vi "Topo & GridSpectr_DriftCorrection_v6.vi"(6 "Internal use":string, 7 "Grid param":T2 {"height (m)" format="%#_6p"; "width (m)" format="%#_6p"; "center Y (m)" format="%#_6p"; "center X (m)" format="%#_6p"}, 8 "Error in (no error)":errorcluster, 9 "Points Y/Index Y":i32, 10 "Points X/Index X":i32, 11 "Method":enum16{"init", "run", "end"}(ring)=enum."end") -> (0 "Error out":errorcluster)   [LabVIEW 2014]
doc: "Example of a measurement VI to be used in the \"Experiments on a Grid\" tool as external VI.\n\nThis example measure the topography and spectroscopy data. The spectroscopy measurements are taken on a subgrid. The data are saved to a sxm and a binary file.\n\n- Nanonis Programming Interface -"
uses:
  <userlib>/Nanonis Prog Interface V5/Nanonis Prog Interface.lvlib
panel:
  out "Images taken":i32=14
  in  "increment":i32=16
  in  "trigger":i32=3 min=1 step=1
  in  "tip Speed (m/s)":sgl=1e-08 format="%.2p"
  in  "Drift Correction 2":T1
  out "X drift":i32
  out "Y drift":i32
  out "Queue Steps":i32=40
  in  "StepsBack":i32=40
  in  "Channel index (0-23)":u8=14
  in  "File name":string="single_mol_shortSTS"
  in  "STS Current":dbl=9.999999717180685e-10 format="%#_6p"
  in  "Imaging Current":dbl=5.00000006675716e-11 format="%#_6p"
  in  "zdrift \nDuration (s)":dbl
  in  "Correct z drift":bool
  out "Status":string="finishing"
  in  "Drift correction Pixels":i32=256 caption="Pixels for drift correction"
  out "Y Offset":dbl
  out "X Offset":dbl
  out "Points taken":dbl=14.0
  in  "Drift Correction every":i32=16
  in  "Y subgrid spacing":u16=1
  in  "X subgrid spacing":u16=1
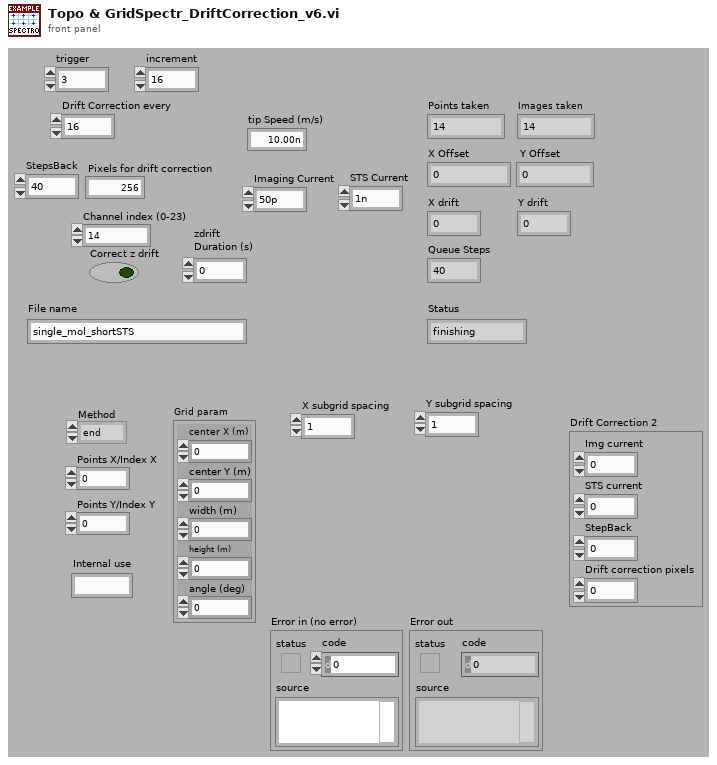
[diagram p1: front panel]
types:
  T1 = cluster{"Img current":dbl, "STS current":dbl, "StepBack":dbl, "Drift correction pixels":dbl}
  T2 = cluster{"center X (m)":sgl, "center Y (m)":sgl, "width (m)":sgl, "height (m)":sgl, "angle (deg)":sgl}
  T3 = cluster{"center X":sgl, "center Y":sgl, "angle":sgl, "width":sgl, "height":sgl, "# pixels":i32, "# lines":i32}
  T4 = cluster{"Name":string, "Calibration":sgl, "Offset":sgl, "Channel index":i32}[]
  T5 = cluster{"up/down":bool, "time/line":sgl, "start time":timestamp, "end time":timestamp}
  T6 = cluster{"Z averaging time (s)":sgl, "Z offset (m)":sgl, "Initial settling time (s)":sgl}
  T7 = cluster{"Max. slew rate (V/s)":sgl, "Settling time (s)":sgl, "Integration time (s)":sgl}
  T8 = cluster{"End settling time (s)":sgl, "Z control time (s)":sgl}
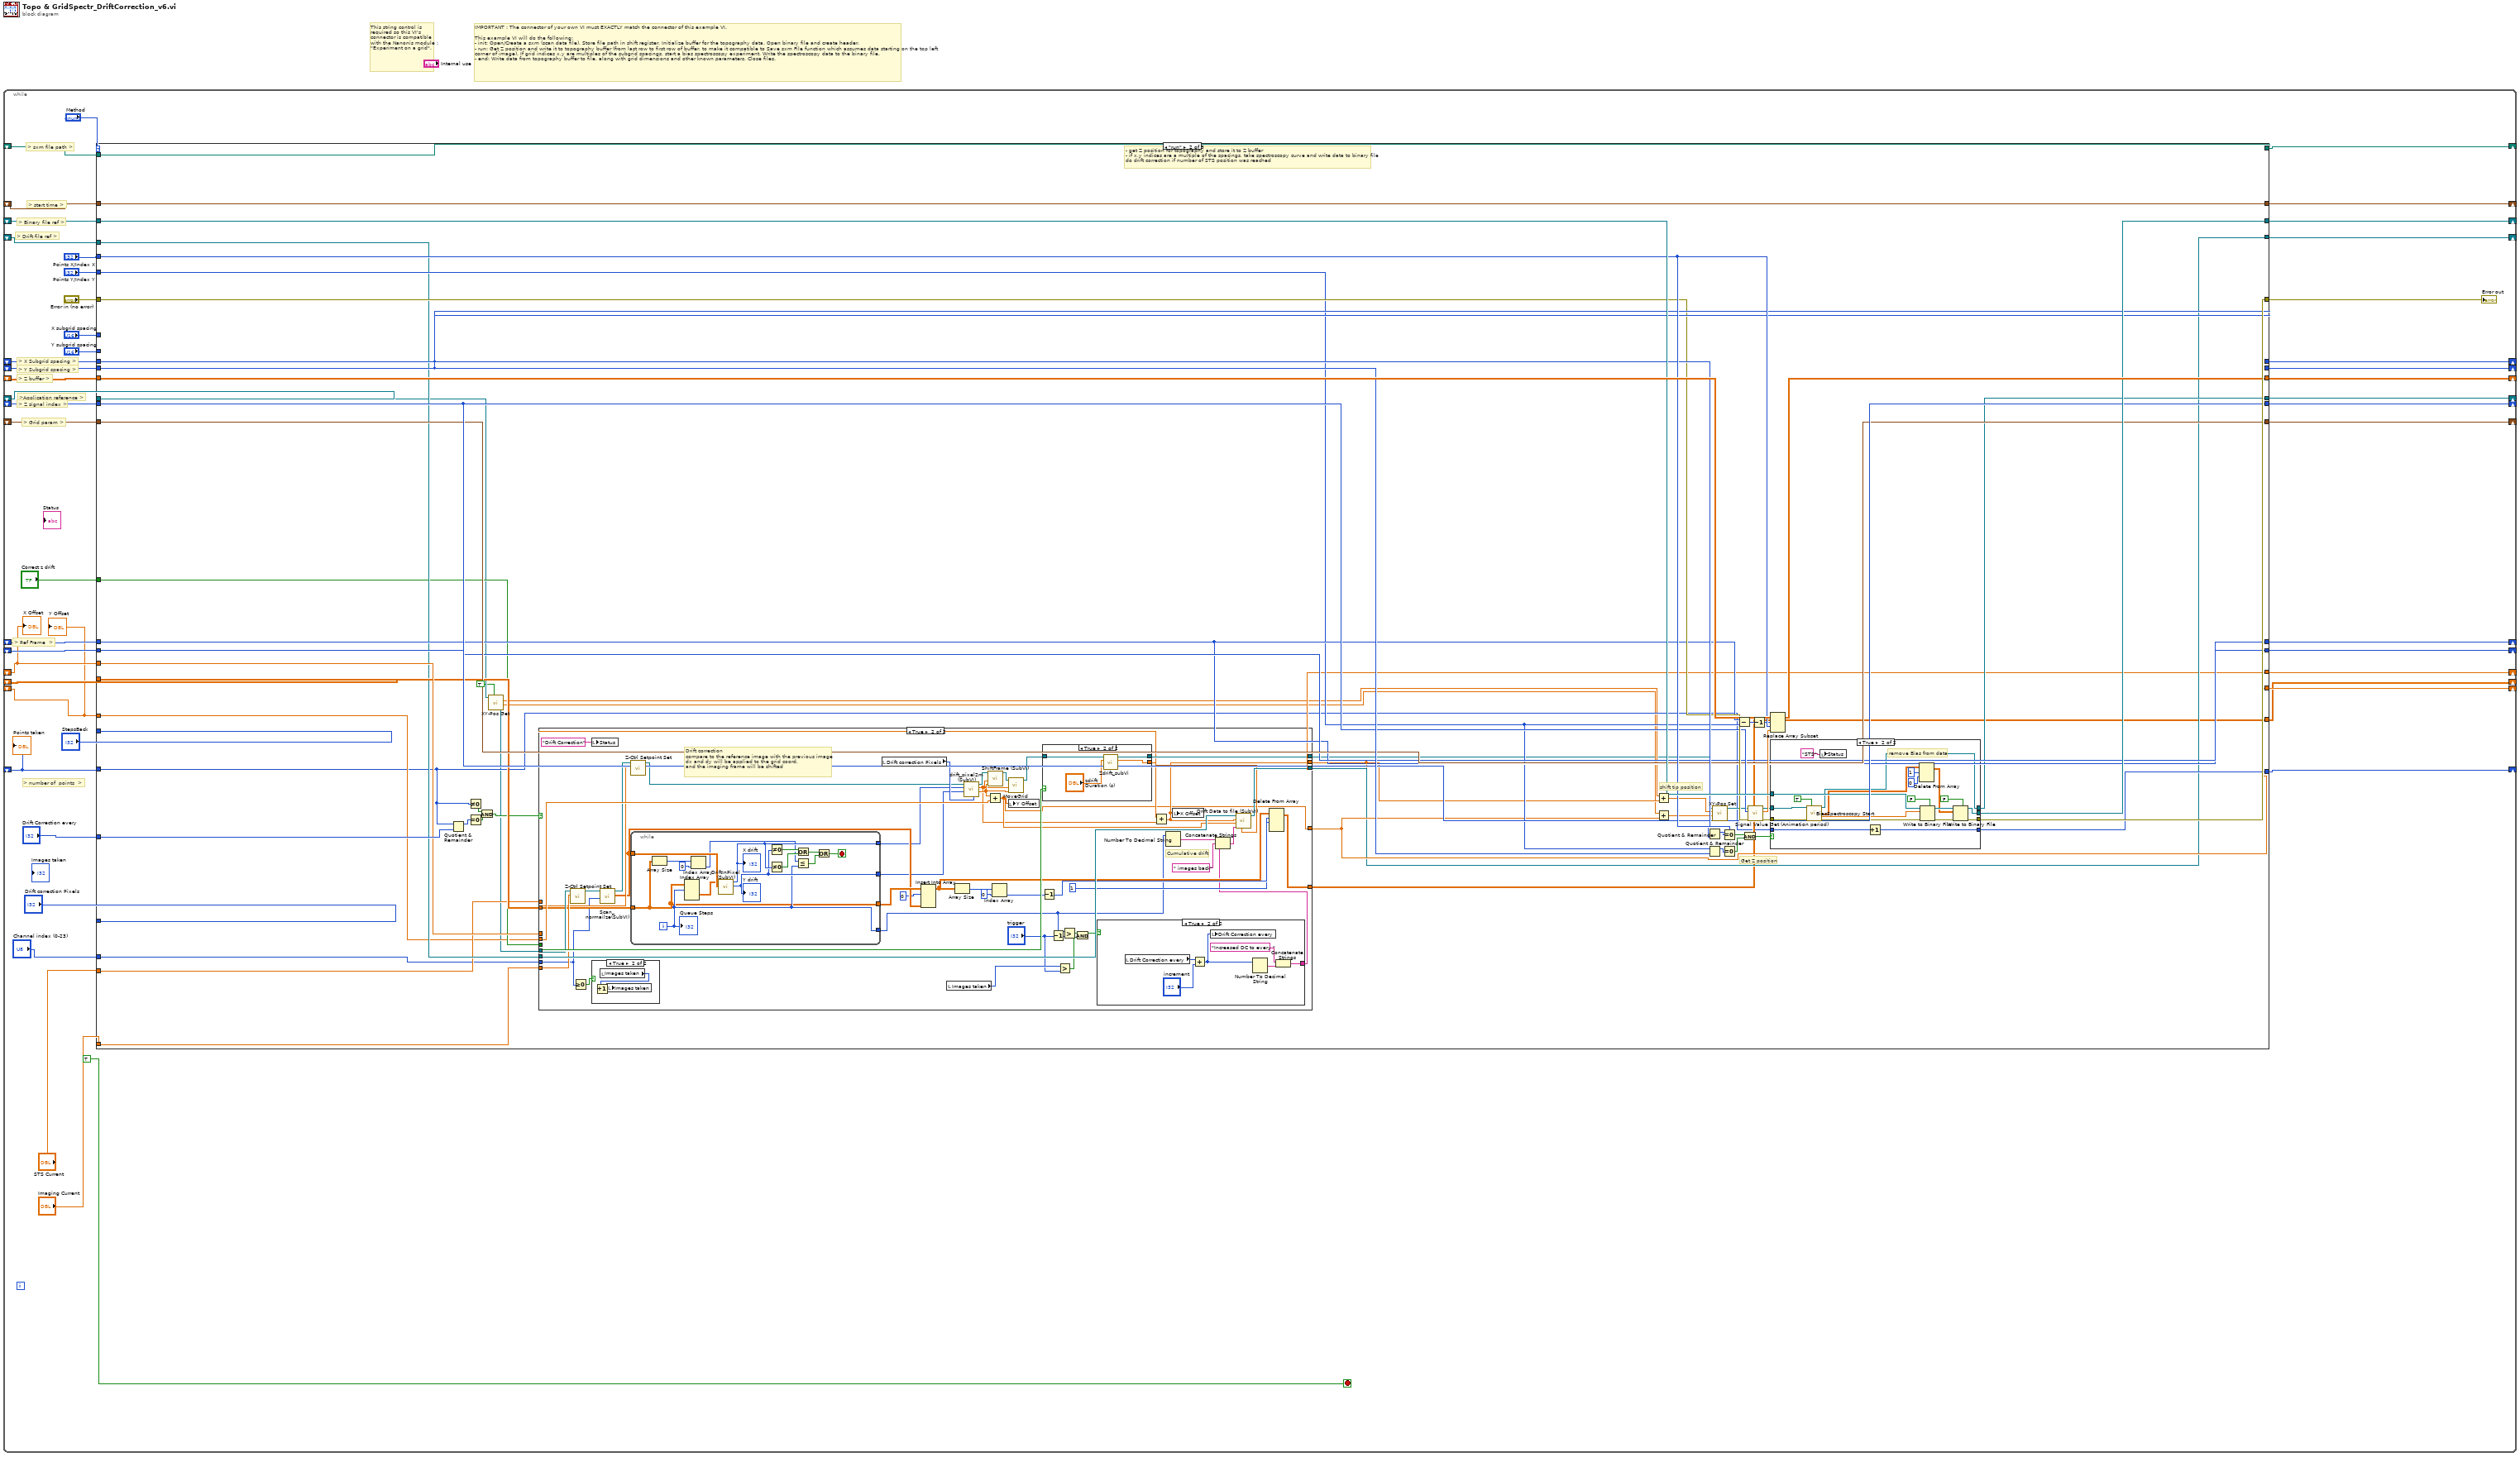
[diagram p0: block diagram]
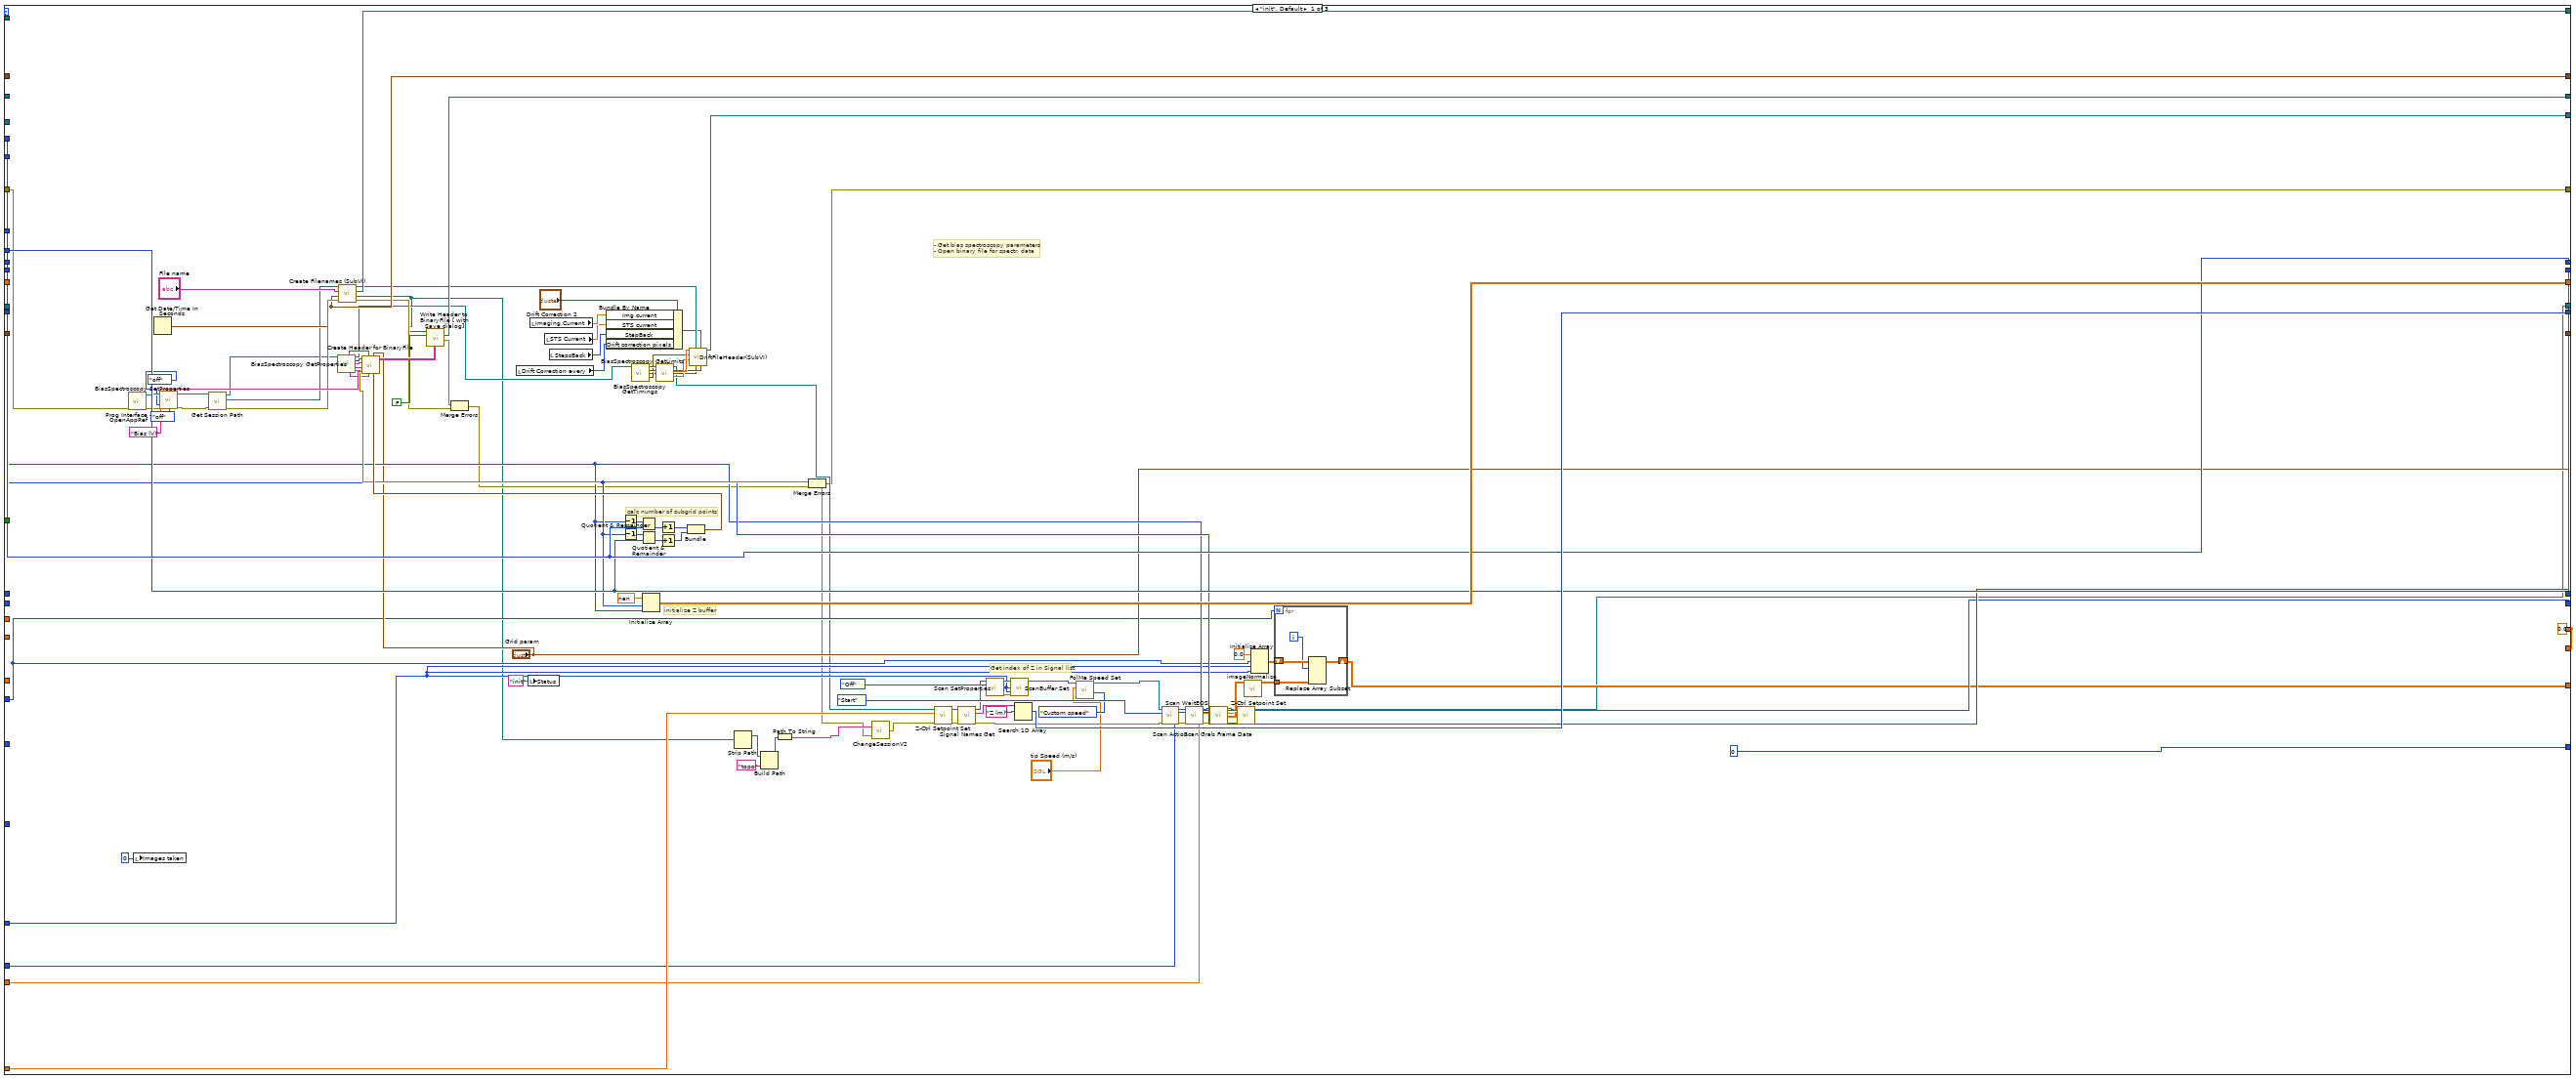
[diagram p2: hidden frame]
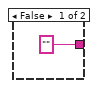
[diagram p5: hidden frame]
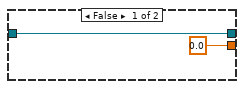
[diagram p6: hidden frame]
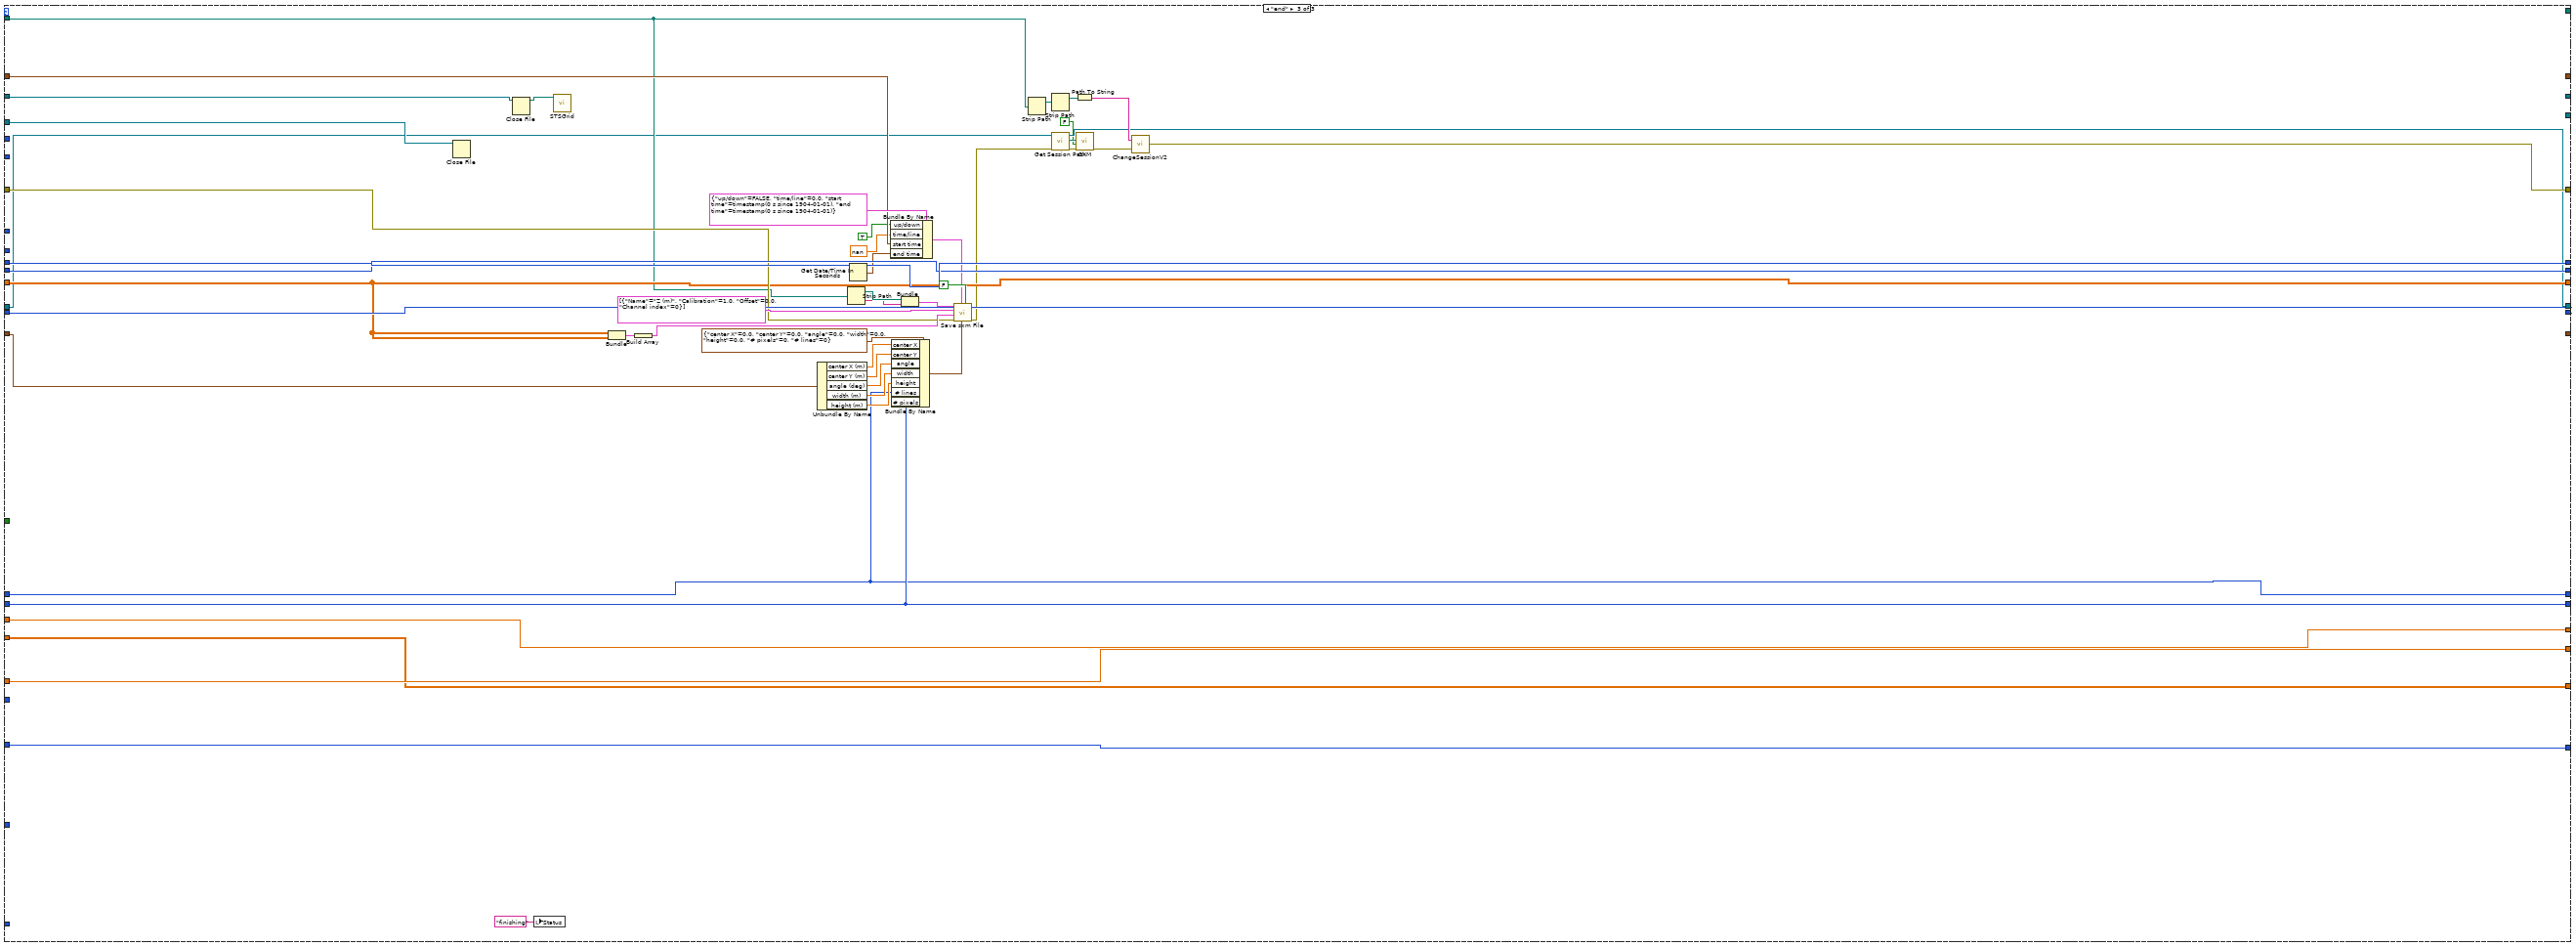
[diagram p8: hidden frame]
diagram:
  # "This string control is required so this VI's connector is compatible with the Nanonis module : \"Experiment on a grid\"."
  # "IMPORTANT : The connector of your own VI must EXACTLY match the connector of this example VI.\n\nThis example VI will do the following:\n- init: Open/Create a sxm (scan data file). Store file path in shift register. Initialize buffer for the topography data. Open binary file and create header.\n- run: Get Z position and write it to topography buffer (from last row to first row of buffer, to make it compatible to Save sxm File function which assumes data starting on the top left corner of image). If grid indices x,y are multiples of the subgrid spacings, start a bias spectroscopy experiment. Write the spectroscopy data to the binary file.\n- end: Write data from topography buffer to file, along with grid dimensions and other known parameters. Close files."
  n1 = while {
    shift-right: [w22] -> _
    shift-left: _ -> [w45]
    shift-right: [w40] -> _
    shift-left: _ -> [w39]
    shift-right: [w37] -> _
    shift-left: _ -> [w38]
    shift-right: [w36] -> _
    shift-left: _ -> [w35]
    shift-right: [w29] -> _
    shift-left: _ -> [w31]
    shift-right: [w30] -> _
    shift-left: _ -> [w32]
    shift-right: [w28] -> _
    shift-left: _ -> [w27]
    shift-right: [w26] -> _
    shift-left: _ -> [w25]
    shift-right: [w24] -> _
    shift-left: _ -> [w23]
    shift-right: [w21] -> _
    shift-left: _ -> [w20]
    shift-right: [w19] -> _
    shift-left: _ -> [w18]
    shift-right: [w17] -> _
    shift-left: _ -> [w10]
    shift-right: [w16] -> _
    shift-left: _ -> [w9]
    shift-right: [w15] -> _
    shift-left: _ -> [w12]
    shift-right: [w14] -> _
    shift-left: _ -> [w11]
    shift-right: [w7] -> _
    shift-left: _ -> [w6]
    stop <- TRUE stop-if-true
    # "> Drift file ref >"
    # "> number of  points  >"
    # "> Ref Frame  >"
    # "> Grid param >"
    # "> start time >"
    # ">Application reference >"
    # "> Y Subgrid spacing >"
    # "> X Subgrid spacing >"
    # "> Z signal index >"
    # "> Binary file ref >"
    # "> Z buffer >"
    # "> sxm file path >"
    n2 = case shown="\"run\"" "Method" {
      tunnel: [w96 w205 _] -> w22
      tunnel: w45 -> [_ w205 w322]
      tunnel: "Error in (no error)" -> [w98 w191 w345]
      tunnel: [w56 w204 w320] -> w43
      tunnel: "Points X/Index X" -> [w122 w199 _]
      tunnel: "Points Y/Index Y" -> [w123 w183 _]
      tunnel: [w146 w202 w334] -> w40
      tunnel: w39 -> [_ w203 w334]
      tunnel: w38 -> [_ w201 w326]
      tunnel: [w138 w200 _] -> w37
      tunnel: [w136 w189 w359] -> w36
      tunnel: w35 -> [_ w189 w359]
      tunnel: "X subgrid spacing" -> [w135 _ _]
      tunnel: "Y subgrid spacing" -> [w134 _ _]
      tunnel: w32 -> [_ w193 w358]
      tunnel: w31 -> [_ w192 w357]
      tunnel: [w135 w193 w358] -> w30
      tunnel: [w134 w192 w357] -> w29
      tunnel: [w69 w175 w316] -> w28
      tunnel: w27 -> [_ w156 w317]
      tunnel: ["Grid param" w186 _] -> w26
      tunnel: w25 -> [_ w186 w344]
      tunnel: [w95 w187 _] -> w24
      tunnel: w23 -> [_ w187 w352]
      tunnel: [w123 w184 w335] -> w21
      tunnel: w20 -> [_ w184 w335]
      tunnel: [w122 w185 w336] -> w19
      tunnel: w18 -> [_ w185 w336]
      tunnel: [w113 w165 w333] -> w17
      tunnel: [w113 w170 w331] -> w16
      tunnel: [w90 w162 w327] -> w15
      tunnel: [0 w180 w332] -> w14
      tunnel: w11 -> [_ w159 w332]
      tunnel: "Drift Correction every" -> [_ w178 _]
      tunnel: w12 -> [_ w169 w327]
      tunnel: w10 -> [_ w176 w333]
      tunnel: w9 -> [_ w160 w331]
      tunnel: "Drift correction Pixels" -> [w89 _ _]
      tunnel: [w85 w167 _] -> w7
      tunnel: w6 -> [_ w168 w328]
      tunnel: "Correct z drift" -> [_ w166 _]
      tunnel: "Imaging Current" -> [w104 w164 _]
      tunnel: "STS Current" -> [w100 w163 _]
      tunnel: "Channel index (0-23)" -> [w93 w161 _]
      tunnel: "StepsBack" -> [w88 _ _]
      frame "init", Default {
        w113 = 0.0
        # "- Get bias spectroscopy parameters\n- Open binary file for spectr. data"
        # "initialize Z buffer"
        # "calc number of subgrid points"
        # "Get index of Z in Signal list"
        n3 = call <userlib>:"Prog Interface - OpenAppRef.vi"("Error in (no error)"=w98) -> ("Error out"=w54:errorcluster, "Application reference"=w99:refnum<vi>)  [unwired: 5 in]
        n4 = local write "Images taken"(0 ("Images taken")) -> ()
        n5 = Get Date/Time In Seconds() -> (seconds since 1Jan1904=w95:timestamp)
        n6 = call <userlib>:"BiasSpectroscopy SetProperties.vi"("Application ref in"=w99, "Autosave (no change)"=enum16{"no change", "on", "off"}."off", "Error in (no error)"=w54, "Save dialog"=enum16{"no change", "on", "off"}."off") -> ("Application ref out"=w50:refnum<vi>, "Error out"=w49:errorcluster)  [unwired: 10 in]
        n7 = call <userlib>:"Get Session Path.vi"("error in (no error)"=w49, "Application ref in"=w50) -> ("error out"=w97:errorcluster, "Session path"=w62:path, "Application ref out"=w51:refnum<vi>)  [unwired: 7 in]
        n8 = call <userlib>:"BiasSpectroscopy GetProperties.vi"("Application ref in"=w51) -> ("Backward sweep"=w142:bool, "Application ref out"=w68:refnum<vi>, "Number of points"=w125:i32, "Channels"=w124:string[], "Parameters"=w140:string[], "Fixed parameters"=w127:string[], "Error out"=w139:errorcluster)  [unwired: 6 in, 2 out]
        n9 = call "Create Filenames (SubVI).vi"("error in (no error)"=w97, "seconds since 1Jan1904"=w95, "File name"="File name", "Session path"=w62) -> ("error out"=w70:errorcluster, "binFilePath"=w58:path, "topoFilePath"=w96:path, "Drift File out"=w86:refnum<file>)  [unwired: 4 in]
        n10 = local read "Drift Correction every"() -> (w80:i32)
        n11 = local write "Status"("init" ("Status")) -> ()
        n12 = local read "Imaging Current"() -> (w82:dbl)
        n13 = local read "STS Current"() -> (w81:dbl)
        n14 = local read "StepsBack"() -> (w79:i32)
        n15 = Bundle By Name(cluster="Drift Correction 2", "Img current"=w82, "STS current"=w81, "StepBack"=w79, "Drift correction pixels"=w80) -> (w83:T1)
        n16 = Decrement(x=w122) -> (x-1=w133:i32)
        n17 = Decrement(x=w123) -> (x-1=w132:i32)
        n18 = call <userlib>:"BiasSpectroscopy GetTimings.vi"("Application ref in"=w68) -> ("Application ref out"=w78:refnum<vi>, "Initialization"=w75:T6, "Sweep Timing"=w73:T7, "End of Sweep"=w74:T8)  [unwired: 10 in, 1 out]
        n19 = Quotient & Remainder(x=w133, y=w135) -> (floor(x/y)=w131:i32)  [unwired: 1 out]
        n20 = Quotient & Remainder(x=w132, y=w134) -> (floor(x/y)=w130:i32)  [unwired: 1 out]
        n21 = Initialize Array(sgl nan ("element"), w123, w122) -> (w146:sgl[][])
        n22 = call <userlib>:"BiasSpectroscopy GetLimits.vi"("Application ref in"=w78) -> ("End value (V)"=w76:sgl, "Start value (V)"=w77:sgl, "Application ref out"=w67:refnum<vi>)  [unwired: 5 in, 1 out]
        n23 = Increment(x=w131) -> (x+1=w129:i32)
        n24 = Increment(x=w130) -> (x+1=w128:i32)
        n25 = Bundle(w129, w128) -> (w141:cluster{i32, i32})  [unwired: 1 in]
        n26 = call <userlib>:"Create Header for BinaryFile.vi"("Grid points"=w141, "Grid param"="Grid param", "Fixed parameters"=w127, "Backward sweep"=w142, "Sweep signal"="Bias (V)" ("Sweep Signal"), "Parameters"=w140, "Channels"=w124, "Points per sweep"=w125) -> ("Header (fixed attributes)"=w144:string[][])  [unwired: 3 in]
        n27 = call <userlib>:"Write Header to BinaryFile [ with Save dialog].vi"("Fixed Attributes"=w144, "Show Dialog? (T)"=FALSE, "Filename"=w58) -> ("Error out"=w71:errorcluster, "File ref"=w138:refnum<file>)  [unwired: 5 in, 2 out]
        n28 = Merge Errors(w71, w70) -> (w72:errorcluster)
        n29 = call "DriftFileHeader(SubVI).vi"("Initialization"=w75, "Drift Correction"=w83, "Sweep Timing"=w73, "Byte Stream File in"=w86, "End value (V)"=w76, "End of Sweep"=w74, "Start value (V)"=w77) -> ("Byte Stream File out"=w85:refnum<file>)  [unwired: 4 in]
        n30 = Strip Path(path=w58) -> (stripped path=w61:path)  [unwired: 1 out]
        n31 = Build Path(base path=w61, name or relative path="topo") -> (appended path=w59:path)
        n32 = Path To String(path=w59) -> (string=w57:string)
        n33 = Merge Errors(w139, w72) -> (w56:errorcluster)
        n34 = call "ChangeSessionV2.vi"("error in (no error)"=w56, "Session"=w57) -> ("error out"=w55:errorcluster)
        n35 = call <userlib>:"Z-Ctrl Setpoint Set.vi"("error in (no error)"=w55, "Z Controller setpoint"=w104, "Application ref in"=w67) -> ("error out"=w103:errorcluster, "Application ref out"=w105:refnum<vi>)  [unwired: 7 in]
        n36 = call <userlib>:"Signal Names Get.vi"("error in (no error)"=w103, "Application ref in"=w105) -> ("error out"=w114:errorcluster, "Signals Names"=w126:string[], "Application ref out"=w109:refnum<vi>)  [unwired: 5 in]
        n37 = call <userlib>:"Scan SetProperties.vi"("Application ref in"=w109, "Continuous scan"=enum16{"No change", "On", "Off"}."Off") -> ("Application ref out"=w111:refnum<vi>, "Error out"=w110:errorcluster)  [unwired: 12 in]
        n38 = call <userlib>:"ScanBuffer Set.vi"("Application ref in"=w111, "Pixels"=w89, "Lines"=w89, "error in (no error)"=w110) -> ("Application ref out"=w66:refnum<vi>)  [unwired: 10 in, 1 out]
        n39 = Search 1D Array(1D array=w126, element="Z (m)") -> (index of element=w136:i32)  [unwired: 1 in]
        n40 = call <userlib>:"FolMe Speed Set.vi"("Speed Setting (Custom)"=enum32{"Scan speed", "Custom speed"}."Custom speed", "Speed (m/s)"="tip Speed (m/s)", "Application ref in"=w66) -> ("Application ref out"=w65:refnum<vi>)  [unwired: 5 in, 1 out]
        n41 = call <userlib>:"Scan Action.vi"("error in (no error)"=w114, "Scan action (Start)"=enum16{"Start", "Stop", "Pause", "Resume"}."Start", "Application ref in"=w65) -> ("error out"=w120:errorcluster, "Application ref out"=w119:refnum<vi>)  [unwired: 6 in]
        n42 = call <userlib>:"Scan WaitEOS.vi"("error in (no error)"=w120, "Application ref in"=w119) -> ("error out"=w117:errorcluster, "Application ref out"=w118:refnum<vi>)  [unwired: 5 in, 2 out]
        n43 = call <userlib>:"Scan Grab Frame Data.vi"("Application ref in"=w118, "Channel index (0-23)"=w93, "error in (no error)"=w117) -> ("Application ref out"=w102:refnum<vi>, "Scan frame data"=w106:sgl[][], "error out"=w101:errorcluster)  [unwired: 8 in, 2 out]
        n44 = call <userlib>:"Z-Ctrl Setpoint Set.vi"("error in (no error)"=w101, "Z Controller setpoint"=w100, "Application ref in"=w102) -> ("Application ref out"=w69:refnum<vi>)  [unwired: 7 in, 1 out]
        n45 = call "imageNormalize.vi"("Data"=w106) -> ("Array"=w87:dbl[][])  [unwired: 10 in]
        n46 = Initialize Array(0.0 ("element"), w88, w89, w89) -> (w91:dbl[][][])
        n47 = for {
          N: w88 -> [_]
          tunnel: w87 -> [w149]
          shift-right: [w148] -> w90
          shift-left: w91 -> [w150]
          i -> [w147]
          n48 = Replace Array Subset(array=w150, new element=w149, index (dim 0)=w147) -> (w148:dbl[][][])  [unwired: 2 in]
        }
      }
      frame "run" {
        # "shift tip position"
        # "Get Z position"
        # "- get Z position for topography and store it to Z buffer\n- if x,y indices are a multiple of the spacings, take spectroscopy curve and write data to binary file\ndo drift correction if number of STS position was reached"
        n49 = Quotient & Remainder(x=w159, y=w178) -> (x-y*floor(x/y)=w179:i32)  [unwired: 1 out]
        n50 = Not Equal To 0?(x=w159) -> (x != 0?=w157:bool)
        n51 = Equal To 0?(x=w179) -> (x = 0?=w177:bool)
        n52 = And(x=w157, y=w177) -> (x .and. y?=w158:bool)
        n53 = call <userlib>:"XY-Pos Get.vi"("Wait for newest data (F=False)"=TRUE, "Application ref in"=w156) -> ("Y (m)"=w152:sgl, "X (m)"=w153:sgl, "Application ref out"=w155:refnum<vi>)  [unwired: 5 in, 1 out]
        n54 = case shown="True" w158 {
          tunnel: w155 -> [w210 w248]
          tunnel: [w210 w254] -> w151
          tunnel: w169 -> [w207 w243]
          tunnel: [w209 w250] -> w165
          tunnel: [w208 w249] -> w170
          tunnel: w176 -> [w209 w252]
          tunnel: w160 -> [w208 w253]
          tunnel: [w207 w236] -> w162
          tunnel: w168 -> [w206 w257]
          tunnel: [w206 w256] -> w167
          tunnel: w166 -> [_ w251]
          tunnel: w164 -> [_ w247]
          tunnel: w163 -> [_ w245]
          tunnel: w161 -> [_ w212]
          frame False {
          }
          frame True {
            # "Cumulative drift"
            # "Drift correction \ncompare to the reference image with the previous image \ndx and dy will be applied to the grid coord, \nand the imaging frame will be shifted"
            n55 = call <userlib>:"Z-Ctrl Setpoint Set.vi"("Z Controller setpoint"=w247, "Application ref in"=w248) -> ("Application ref out"=w244:refnum<vi>)  [unwired: 8 in, 1 out]
            n56 = Greater Or Equal To 0?(x=w212) -> (x >= 0?=w211:bool)
            n57 = local write "Status"("Drift Correction" ("Status")) -> ()
            n58 = case shown="True" w211 {
              frame False {
              }
              frame True {
                n59 = local read "Images taken"() -> (w260:i32)
                n60 = Increment(x=w260) -> (x+1=w259:i32)
                n61 = local write "Images taken"(w259) -> ()
              }
            }
            n62 = call "Scan_normailze(SubVI).vi"("Channel index (0-23)"=w212, "Application in"=w244) -> ("Array"=w238:dbl[][], "Application out"=w246:refnum<vi>)  [unwired: 7 in, 1 out]
            n63 = call <userlib>:"Z-Ctrl Setpoint Set.vi"("Z Controller setpoint"=w245, "Application ref in"=w246) -> ("Application ref out"=w226:refnum<vi>)  [unwired: 8 in, 1 out]
            n64 = while {
              tunnel: w238 -> [w279]
              tunnel: w243 -> [w269]
              tunnel: [w278] -> w222
              tunnel: [w277] -> w221
              tunnel: [w273] -> w220
              tunnel: [w269] -> w239
              i -> [w273]
              stop <- w275 stop-if-true
              n65 = Array Size(array=w269) -> (size(s)=w272:i32[])
              n66 = Index Array(array=w269, index (dim 0)=w273) -> (element=w268:dbl[][])  [unwired: 2 in]
              n67 = Index Array(array=w272, index=0) -> (element=w270:i32)
              n68 = call "DriftInPixel (SubVI).vi"("New image"=w279, "Ref image"=w268) -> ("Y drift"=w277:i32, "X drift"=w278:i32)  [unwired: 7 in, 1 out]
              "Y drift" <- w277
              "X drift" <- w278
              n69 = Not Equal To 0?(x=w277) -> (x != 0?=w281:bool)
              n70 = Not Equal To 0?(x=w278) -> (x != 0?=w280:bool)
              n71 = Or(x=w281, y=w280) -> (x .or. y?=w276:bool)
              n72 = Less Or Equal?(x=w270, y=w273) -> (x <= y?=w274:bool)
              n73 = Or(x=w276, y=w274) -> (x .or. y?=w275:bool)
              "Queue Steps" <- w273
            }
            n74 = local read "Drift correction Pixels"() -> (w227:i32)
            n75 = Insert Into Array(array=w239, index (dim 0)=0 ("index (page)"), new element=w238) -> (w235:dbl[][][])  [unwired: 2 in]
            n76 = local read "Images taken"() -> (w215:i32)
            n77 = Array Size(array=w235) -> (size(s)=w234:i32[])
            n78 = call "drift_pixel2m (SubVI).vi"("Application in"=w226, "X drift"=w222, "Y drift"=w221, "Drift correction Pixels"=w227) -> ("Application out"=w225:refnum<vi>, "x drift"=w223:sgl, "y drift"=w224:sgl)  [unwired: 2 in, 1 out]
            n79 = Add(x=w224, y=w253) -> (x+y=w249:dbl)
            n80 = call "ShiftFrame (SubVI).vi"("Y shift"=w224, "X shift"=w223, "Application in"=w225) -> ("Application out"=w229:refnum<vi>)  [unwired: 8 in]
            n81 = Index Array(array=w234, index=0) -> (element=w232:i32)
            n82 = call "MoveGrid.vi"("y"=w224, "x"=w223, "Application ref in"=w229) -> ("Application ref out"=w228:refnum<vi>)  [unwired: 7 in, 1 out]
            n83 = local write "Y Offset"(w249) -> ()
            n84 = Decrement(x=w232) -> (x-1=w231:i32)
            n85 = case shown="True" w251 {
              tunnel: [0.0 ("z drift") w287] -> w255
              tunnel: w228 -> [w282 w286]
              tunnel: [w282 w285] -> w254
              frame False {
              }
              frame True {
                n86 = call "Zdrift_subVi.vi"("Duration"="zdrift \nDuration (s)", "Application in"=w286) -> ("z drift"=w287:dbl, "Application out"=w285:refnum<vi>)  [unwired: 7 in, 1 out]
              }
            }
            n87 = Decrement(x="trigger") -> (x-1=w219:i32)
            n88 = Greater?(x=w215, y="trigger") -> (0:w213:bool)
            n89 = Greater?(x=w220, y=w219) -> (0:w217:bool)
            n90 = And(x=w217, y=w213) -> (x .and. y?=w216:bool)
            n91 = case shown="True" w216 {
              tunnel: ["" w262] -> w218
              frame False {
              }
              frame True {
                n92 = local read "Drift Correction every"() -> (w267:i32)
                n93 = Add(x=w267, y="increment") -> (x+y=w265:i32)
                n94 = local write "Drift Correction every"(w265) -> ()
                n95 = Number To Decimal String(number=w265) -> (decimal integer string=w264:string)  [unwired: 1 in]
                n96 = Concatenate Strings("Increased DC to every " ("string"), w264) -> (w262:string)
              }
            }
            n97 = Add(x=w252, y=w223) -> (x+y=w250:dbl)
            n98 = Number To Decimal String(number=w220) -> (decimal integer string=w242:string)  [unwired: 1 in]
            n99 = local write "X Offset"(w250) -> ()
            n100 = Concatenate Strings(w242, " images back" ("string"), w218) -> (w241:string)
            n101 = call "Drift Data to file (SubVI).vi"("z drift"=w255, "Comment"=w241, "y Drift"=w249, "X drift"=w250, "Byte Stream File in"=w257) -> ("Byte Stream File out"=w256:refnum<file>)  [unwired: 6 in]
            n102 = Delete From Array(array=w235, length=1, index (dim 0)=w231) -> (array with subset deleted=w236:dbl[][][])  [unwired: 2 in, 1 out]
          }
        }
        n103 = Add(x=w153, y=w165) -> (x+y=w172:dbl)
        n104 = Add(x=w152, y=w170) -> (x+y=w171:dbl)
        n105 = Quotient & Remainder(x=w199, y=w193) -> (x-y*floor(x/y)=w198:i32)  [unwired: 1 out]
        n106 = Quotient & Remainder(x=w183, y=w192) -> (x-y*floor(x/y)=w197:i32)  [unwired: 1 out]
        n107 = call <userlib>:"XY-Pos Set.vi"("Y (m)"=w171, "X (m)"=w172, "Application ref in"=w151) -> ("Application ref out"=w173:refnum<vi>)  [unwired: 5 in, 1 out]
        n108 = Equal To 0?(x=w198) -> (x = 0?=w196:bool)
        n109 = Equal To 0?(x=w197) -> (x = 0?=w195:bool)
        n110 = Subtract(x=w184, y=w183) -> (x-y=w182:i32)
        n111 = And(x=w196, y=w195) -> (x .and. y?=w194:bool)
        n112 = call <userlib>:"Signal Value Get (Animation period).vi"("error in (no error)"=w191, "Signal index (0-47)"=w189, "Application ref in"=w173) -> ("error out"=w190:errorcluster, "Signal value"=w188:sgl, "Application ref out"=w174:refnum<vi>)  [unwired: 5 in]
        n113 = Decrement(x=w182) -> (x-1=w181:i32)
        n114 = Replace Array Subset(array=w203, new element=w188, index (row)=w181, index (col)=w199) -> (w202:sgl[][])
        n115 = case shown="True" w194 {
          tunnel: [w290 w295] -> w204
          tunnel: w201 -> [w291 w311]
          tunnel: [w291 w309] -> w200
          tunnel: w190 -> [w290 w308]
          tunnel: w174 -> [w289 w300]
          tunnel: [w289 w299] -> w175
          tunnel: [w288 w293] -> w180
          tunnel: w159 -> [w288 w294]
          frame False {
            # "Point indices aren't multiple of subgrid spacing\n=> no spectroscopy at this point"
          }
          frame True {
            # "remove Bias from data"
            n116 = call <userlib>:"BiasSpectroscopy Start.vi"("Application ref in"=w300, "Get data (F)"=TRUE ("Get Data (F)"), "Error in (no error)"=w308) -> ("Application ref out"=w299:refnum<vi>, "Data"=w307:sgl[][], "Parameters"=w306:sgl[], "Error out"=w297:errorcluster)  [unwired: 8 in, 1 out]
            n117 = local write "Status"("STS" ("Status")) -> ()
            n118 = Increment(x=w294) -> (x+1=w293:i32)
            n119 = Delete From Array(array=w307, length=1, index (row)=0 ("index")) -> (array with subset deleted=w305:sgl[][])  [unwired: 1 in, 1 out]
            n120 = Write to Binary File(file (use dialog)=w311, data=w306, error in=w297, 5:FALSE ("prepend array or string size? (T)")) -> (refnum out=w310:refnum<file>, error out=w296:errorcluster)  [unwired: 2 in, 1 out]
            n121 = Write to Binary File(file (use dialog)=w310, data=w305, error in=w296, 5:FALSE ("prepend array or string size? (T)")) -> (refnum out=w309:refnum<file>, error out=w295:errorcluster)  [unwired: 2 in, 1 out]
          }
        }
      }
      frame "end" {
        n122 = Close File(refnum=w328) -> ()  [unwired: 1 in, 2 out]
        n123 = Close File(refnum=w326) -> (path=w325:path)  [unwired: 1 in, 1 out]
        n124 = local write "Status"("finishing" ("Status")) -> ()
        n125 = call "STSGrid.vi"("Binary Spectroscopy File"=w325) -> ()  [unwired: 11 in]
        n126 = Bundle(w334, w334) -> (w356:cluster{sgl[][], sgl[][]})  [unwired: 1 in]
        n127 = Build Array(w356) -> (w355:cluster{sgl[][], sgl[][]}[])
        n128 = Unbundle By Name(w344) -> ("center X (m)"=w342:sgl, "center Y (m)"=w341:sgl, "angle (deg)"=w340:sgl, "width (m)"=w339:sgl, "height (m)"=w338:sgl)
        n129 = Strip Path(path=w322) -> (stripped path=w348:path, name=w347:string)
        n130 = Get Date/Time In Seconds() -> (seconds since 1Jan1904=w330:timestamp)
        n131 = Bundle By Name(cluster=T5 {"up/down"=FALSE, "time/line"=0.0, "start time"=timestamp(0 s since 1904-01-01), "end time"=timestamp(0 s since 1904-01-01)} ("Scan param"), "up/down"=TRUE, "time/line"=sgl nan ("input 7"), "start time"=w352, "end time"=w330) -> (w351:T5)
        n132 = Bundle By Name(cluster=T3 {"center X"=0.0, "center Y"=0.0, "angle"=0.0, "width"=0.0, "height"=0.0, "# pixels"=0, "# lines"=0} ("Scanfield"), "center X"=w342, "center Y"=w341, "angle"=w340, "width"=w339, "height"=w338, "# lines"=w335, "# pixels"=w336) -> (w337:T3)
        n133 = Bundle("stripped path"=w348, "name"=w347) -> (w346:cluster{"stripped path":path, "name":string})  [unwired: 1 in]
        n134 = call <userlib>:"Save sxm File.vi"("Auto file naming? (T)"=FALSE, "Scanfield"=w337, "Scan param"=w351, "error in (no error)"=w345, "Channels data"=w355, "Channels config"=T4 [{"Name"="Z (m)", "Calibration"=1.0, "Offset"=0.0, "Channel index"=0}], "Filename control"=w346) -> ("error out"=w318:errorcluster)  [unwired: 2 in, 2 out]
        n135 = Strip Path(path=w322) -> (stripped path=w324:path)  [unwired: 1 out]
        n136 = Strip Path(path=w324) -> (stripped path=w323:path)  [unwired: 1 out]
        n137 = call <userlib>:"Get Session Path.vi"("error in (no error)"=w318, "Application ref in"=w317) -> ("error out"=w313:errorcluster, "Session path"=w315:path, "Application ref out"=w316:refnum<vi>)  [unwired: 7 in]
        n138 = Path To String(path=w323) -> (string=w319:string)
        n139 = call "SXM.vi"("Path"=w315, "Delete"=FALSE, "error in"=w313) -> ("error out"=w312:errorcluster)  [unwired: 7 in]
        n140 = call "ChangeSessionV2.vi"("error in (no error)"=w312, "Session"=w319) -> ("error out"=w320:errorcluster)
      }
    }
    "Error out" <- w43
    "Points taken" <- w11
    "X Offset" <- w10
    "Y Offset" <- w9
  }
